vi "Ooi Wei Hong TP065329 Client.vi"() -> ()   [LabVIEW 2023]
uses:
  Control 1.ctl
panel:
  in  "Tab Control":enum32{"Login", "Main"}(tab)
  in  "Request":bool
  out "Password Input":string
  in  "Password":T1
  in  "Reveal":bool
  in  "System Close":bool
  in  "Alarm 1":bool
  in  "Alarm 2":bool
  in  "Alarm 3":bool
  in  "Alarm 4":bool
  in  "Alarm 5":bool
  in  "Alarm 6":bool
  in  "Bypass 1":bool
  in  "Bypass 2":bool
  in  "Bypass 3":bool
  in  "Bypass 4":bool
  in  "Bypass 5":bool
  in  "Bypass 6":bool
  in  "Tamper 1":bool
  in  "Tamper 2":bool
  in  "Tamper 3":bool
  in  "Tamper 4":bool
  in  "Tamper 5":bool
  in  "Tamper 6":bool
  in  "Logout quit":bool
  out "Passcode":string
  # "Vilantguard Technologies Security System"
  # "Alarm Switches"
  # "Bypass Switches"
  # "Tamper Switches"
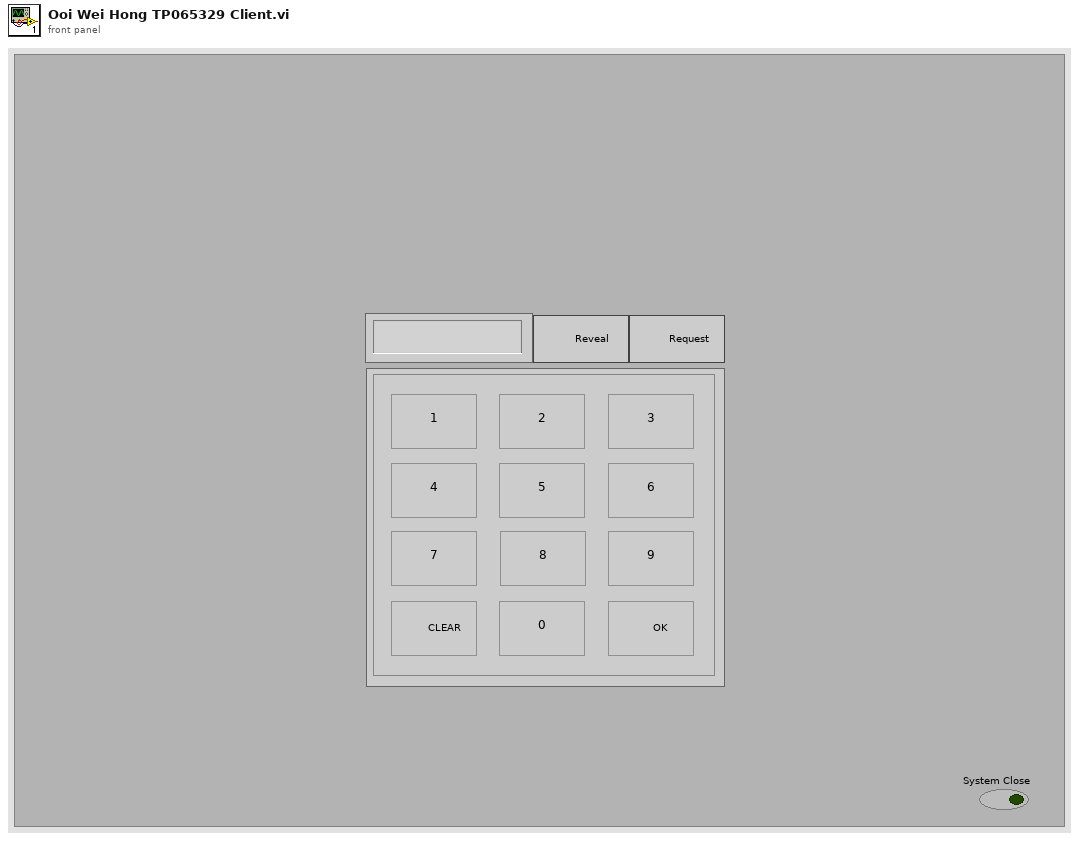
[diagram p1: front panel]
types:
  T1 = cluster{"1":bool, "4":bool, "7":bool, "8":bool, "9":bool, "5":bool, "6":bool, "2":bool, "3":bool, "0":bool, "Previous":bool, "ok":bool}
  T2 = enum8{"Enabled", "Disabled", "Disabled and Grayed Out"}
  T3 = typedef "Control 1.ctl" = enum16{"Init", "Wait", "Zone 1", "Zone 2", "Zone 3", "Zone 4", "Zone 5", "Zone 6"}
  T4 = enum16{"Init", "Wait", "Zone 1", "Zone 2", "Zone 3", "Zone 4", "Zone 5", "Zone 6", "Transmit", "Logging"}
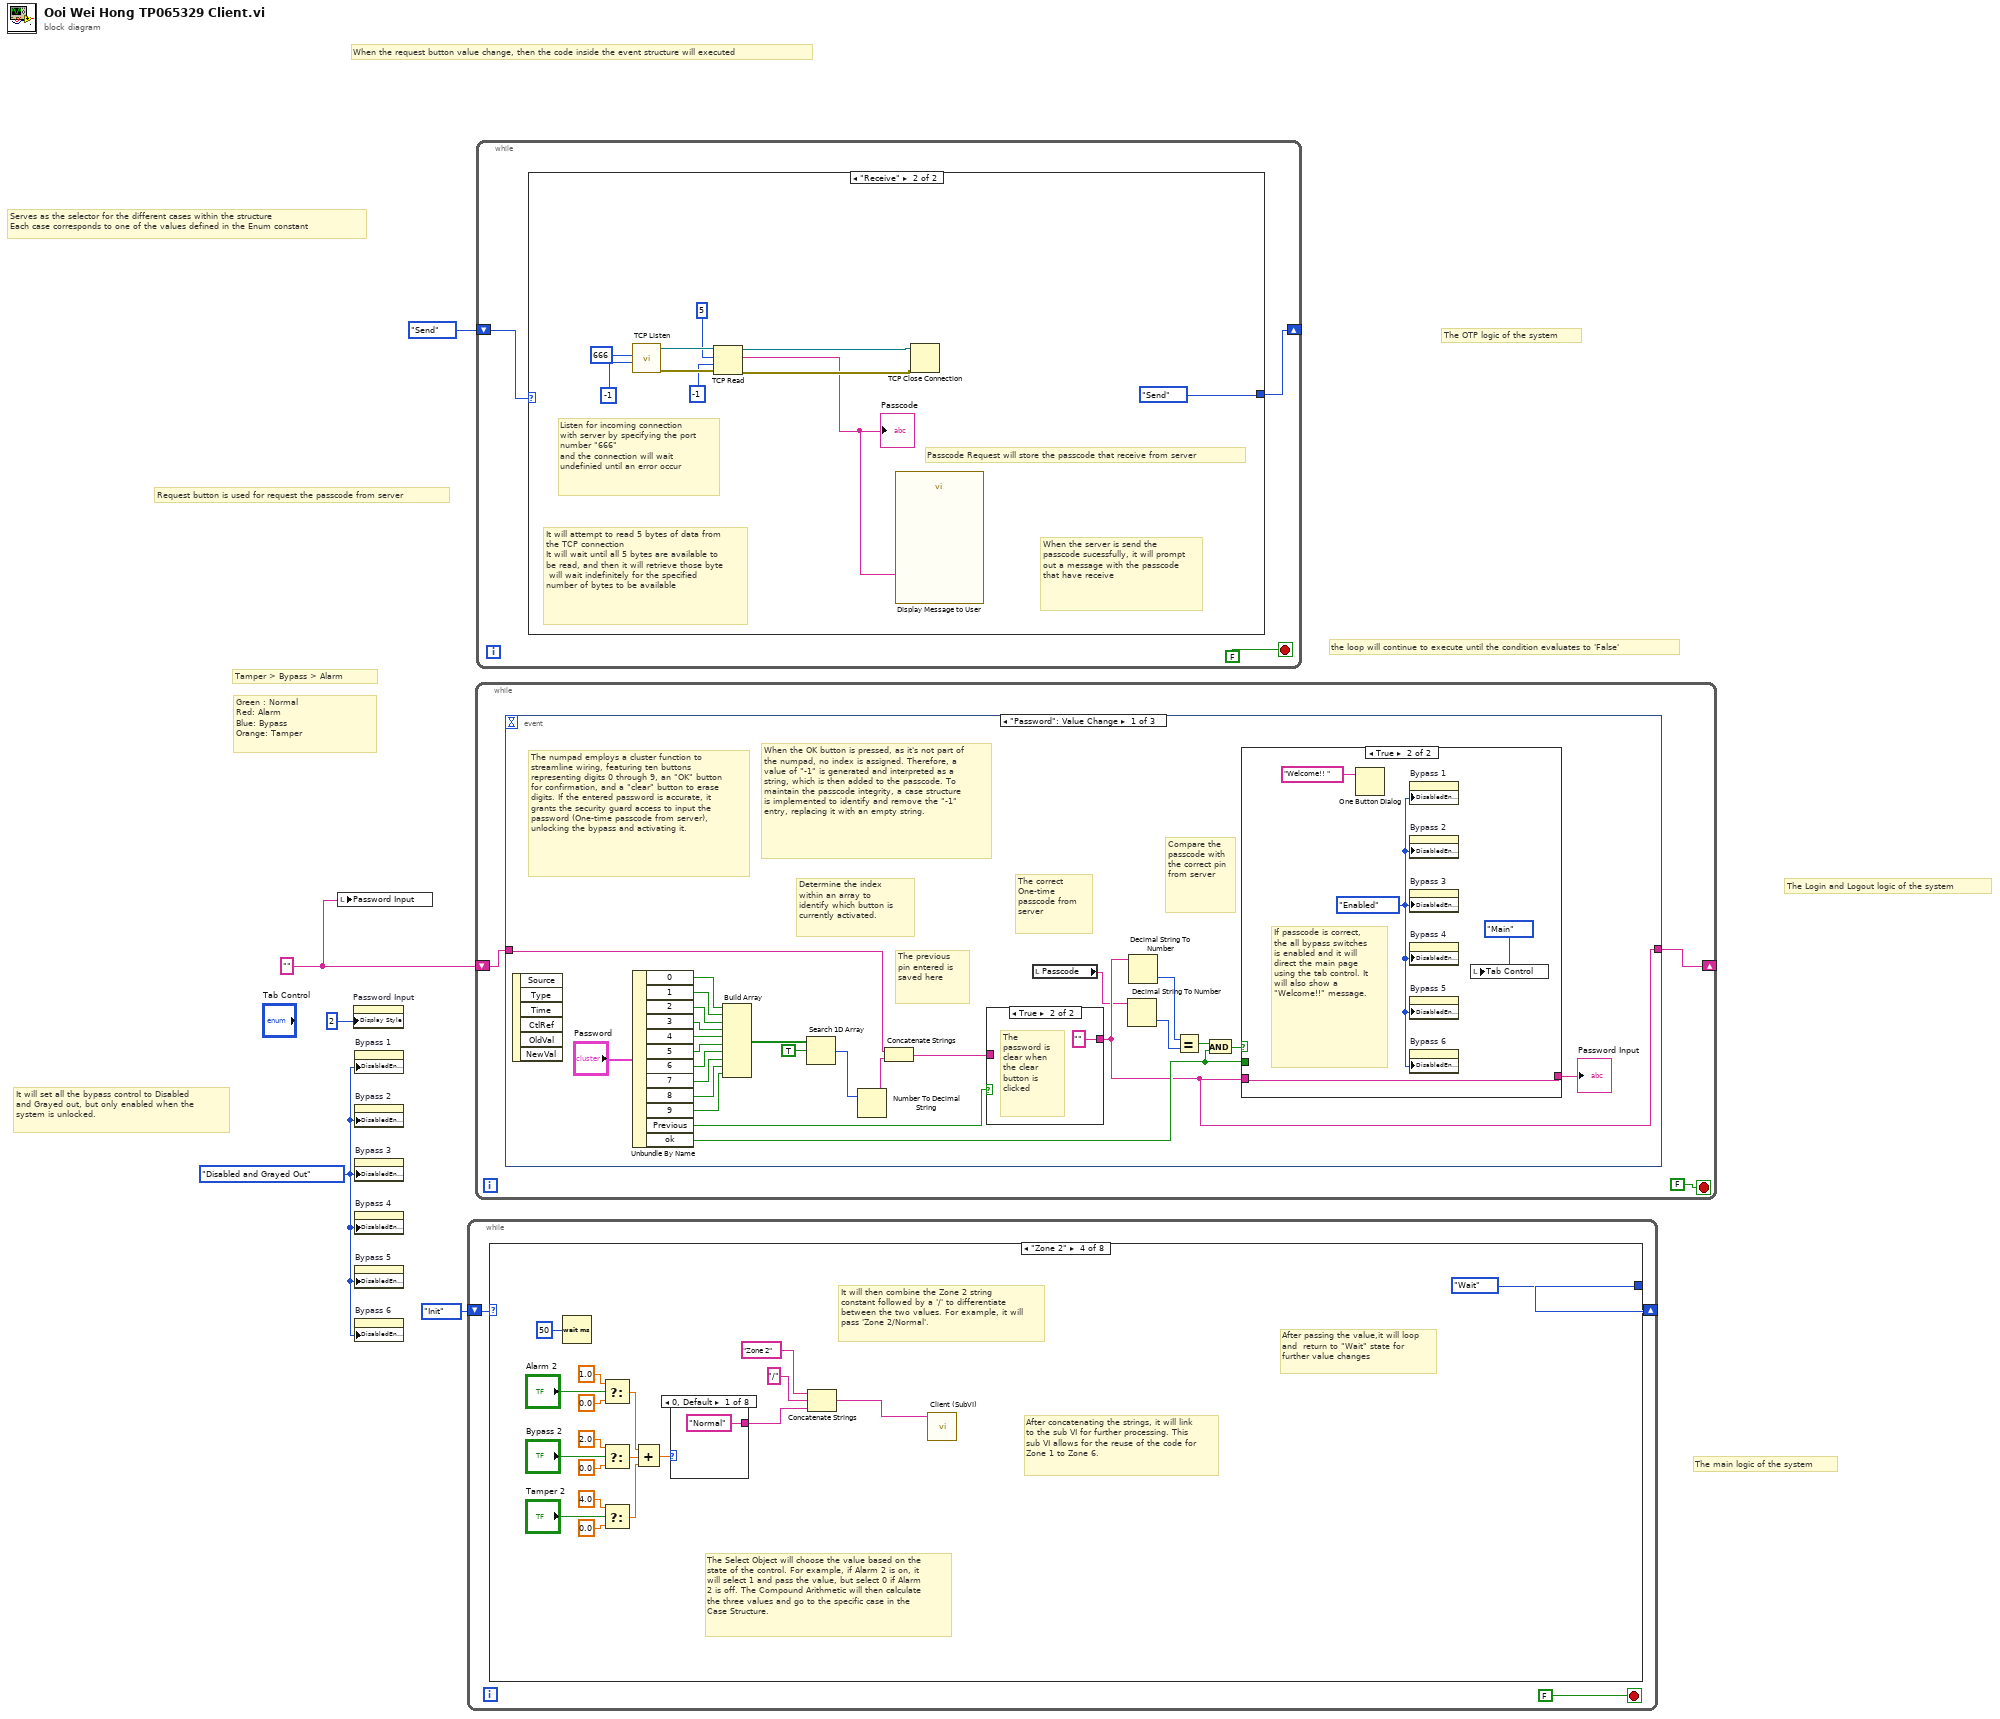
[diagram p0: block diagram]
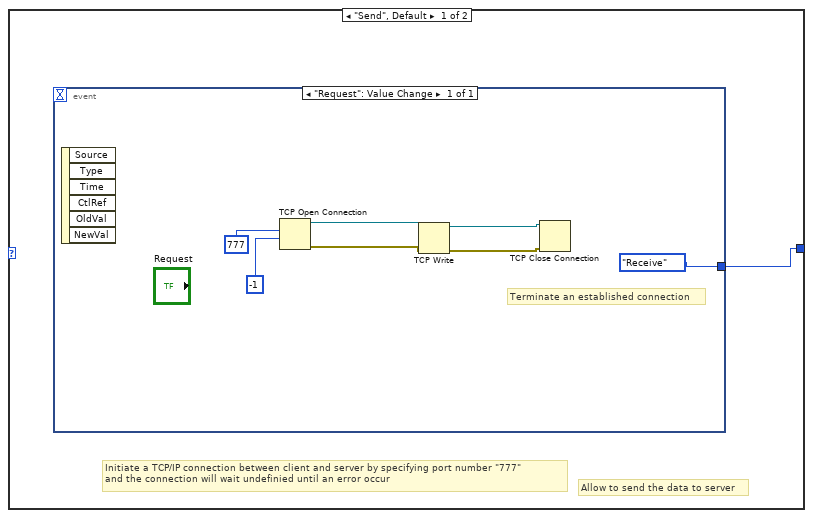
[diagram p2: hidden frame]
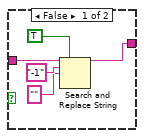
[diagram p3: hidden frame]
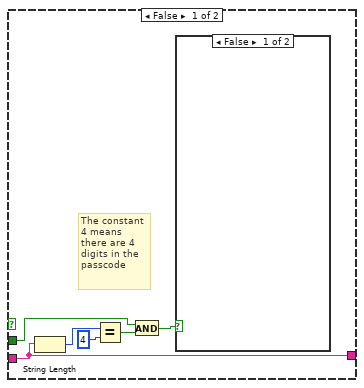
[diagram p4: hidden frame]
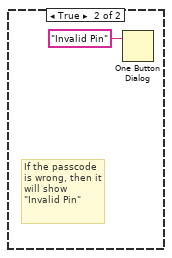
[diagram p5: hidden frame]
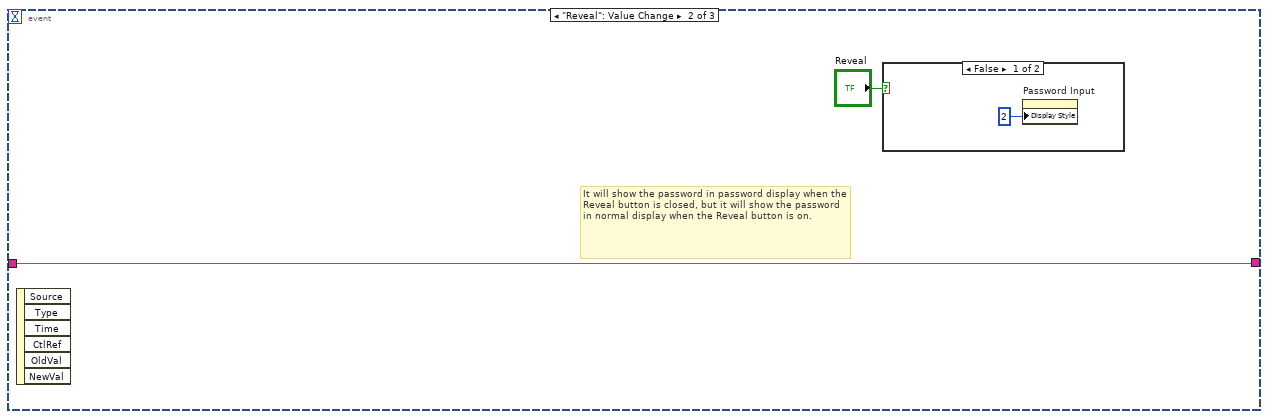
[diagram p6: hidden frame]
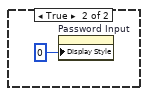
[diagram p7: hidden frame]
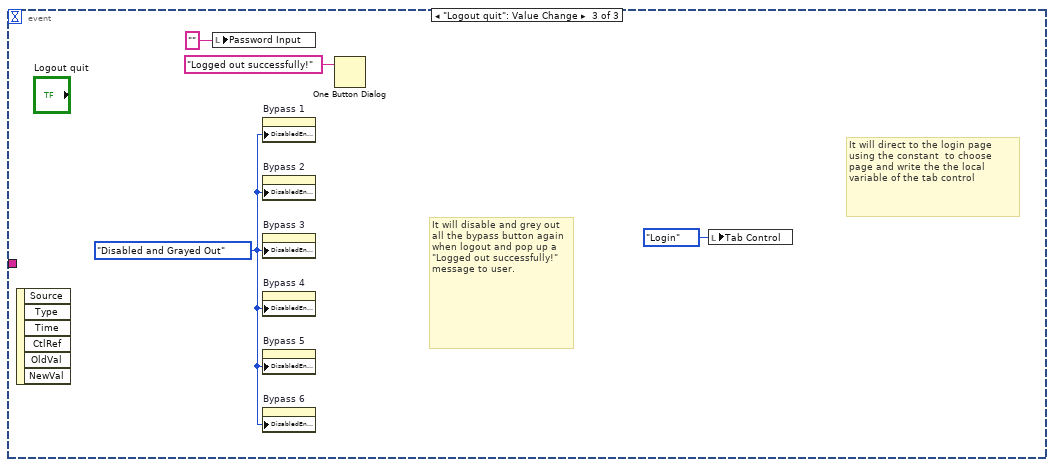
[diagram p8: hidden frame]
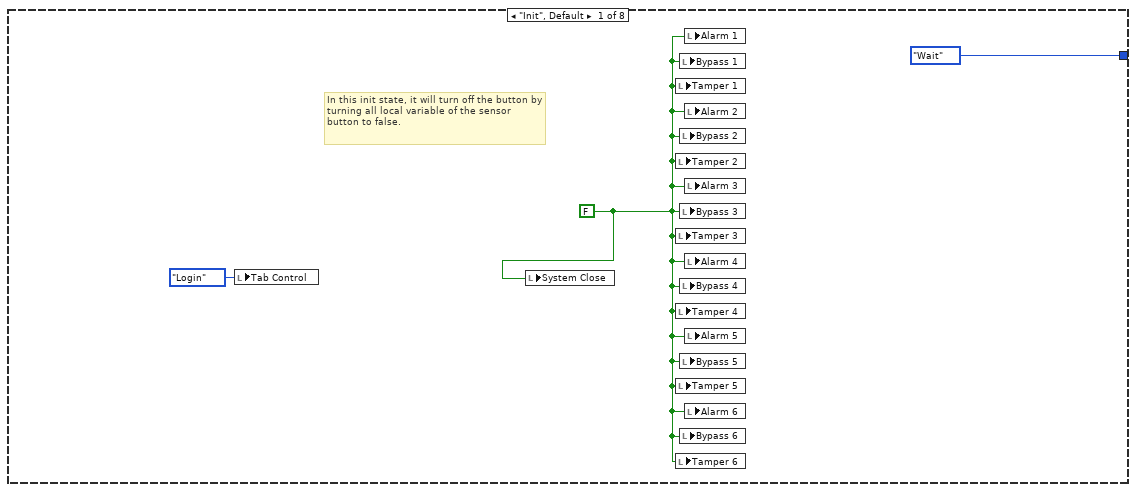
[diagram p9: hidden frame]
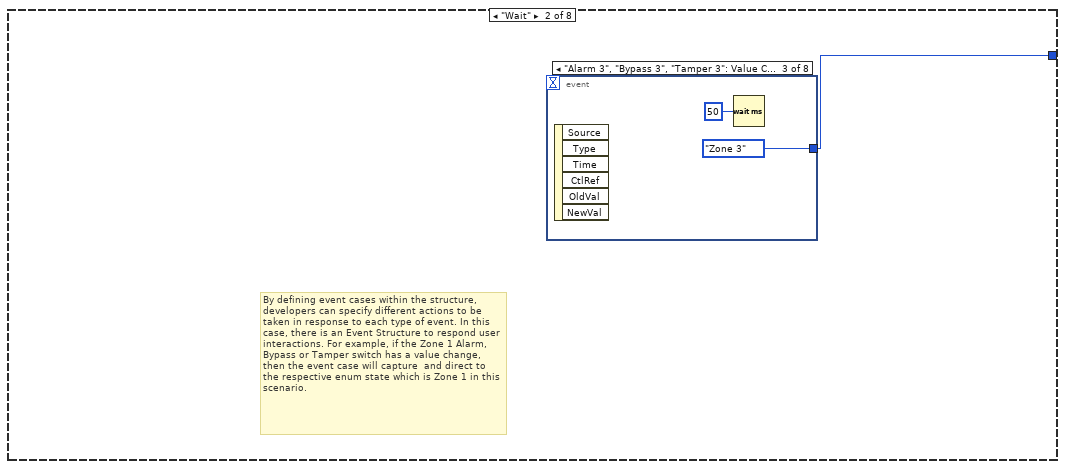
[diagram p10: hidden frame]
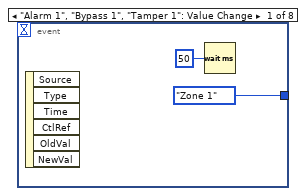
[diagram p11: hidden frame]
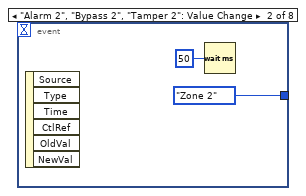
[diagram p12: hidden frame]
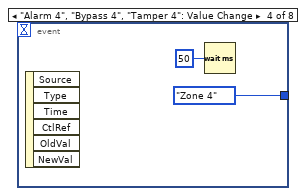
[diagram p13: hidden frame]
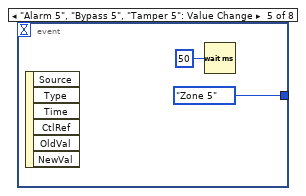
[diagram p14: hidden frame]
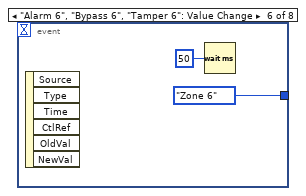
[diagram p15: hidden frame]
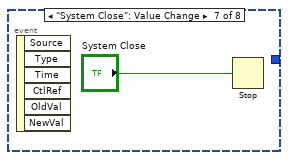
[diagram p16: hidden frame]
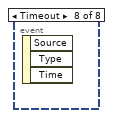
[diagram p17: hidden frame]
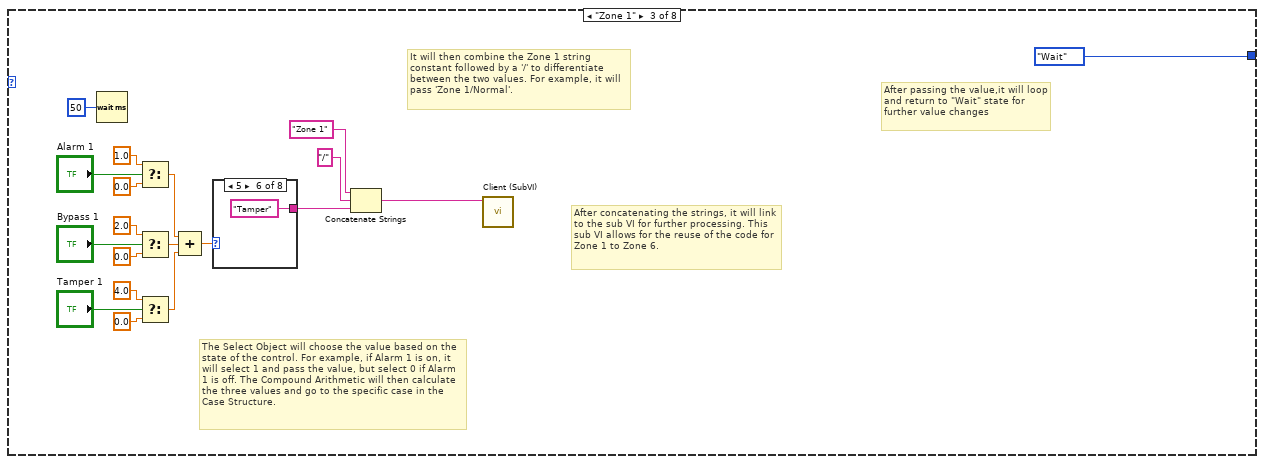
[diagram p18: hidden frame]
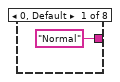
[diagram p19: hidden frame]
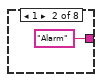
[diagram p20: hidden frame]
diagram:
  w3 = ""
  w4 = T2."Disabled and Grayed Out" ("Disabled")
  # "the loop will continue to execute until the condition evaluates to 'False'"
  # "Request button is used for request the passcode from server"
  # "Serves as the selector for the different cases within the structure\nEach case corresponds to one of the values defined in the Enum constant"
  # "When the request button value change, then the code inside the event structure will executed"
  # "The OTP logic of the system"
  # "The Login and Logout logic of the system"
  # "It will set all the bypass control to Disabled and Grayed out, but only enabled when the system is unlocked."
  # "The main logic of the system"
  # "Green : Normal\nRed: Alarm\nBlue: Bypass\nOrange: Tamper"
  # "Tamper > Bypass > Alarm"
  n1 = local write "Password Input"(w3) -> ()
  n2 = property on="Password Input" class="Str"("Display Style"=u32 2) -> ()  [unwired: 2 in, 2 out]
  n3 = property on="Bypass 1" class="Bool (strict)"("DisabledEnum"=w4) -> ()  [unwired: 2 in, 2 out]
  n4 = property on="Bypass 2" class="Bool (strict)"("DisabledEnum"=w4) -> ()  [unwired: 2 in, 2 out]
  n5 = property on="Bypass 3" class="Bool (strict)"("DisabledEnum"=w4) -> ()  [unwired: 2 in, 2 out]
  n6 = property on="Bypass 4" class="Bool (strict)"("DisabledEnum"=w4) -> ()  [unwired: 2 in, 2 out]
  n7 = property on="Bypass 5" class="Bool (strict)"("DisabledEnum"=w4) -> ()  [unwired: 2 in, 2 out]
  n8 = property on="Bypass 6" class="Bool (strict)"("DisabledEnum"=w4) -> ()  [unwired: 2 in, 2 out]
  n9 = while {
    shift-right: [w8] -> _
    shift-left: Control_1."Init" -> [w7]
    stop <- FALSE stop-if-true
    n10 = case shown="\"Zone 2\"" w7 {
      tunnel: [T4."Wait" w12 Control_1."Wait" Control_1."Wait" Control_1."Wait" Control_1."Wait" Control_1."Wait" Control_1."Wait"] -> w8
      frame "Init", Default {
        w10 = FALSE
        # "In this init state, it will turn off the button by turning all local variable of the sensor button to false."
        n11 = local write "Tab Control"(enum32{"Login", "Main"}."Login" ("Tab Control")) -> ()
        n12 = local write "System Close"(w10) -> ()
        n13 = local write "Tamper 1"(w10) -> ()
        n14 = local write "Tamper 2"(w10) -> ()
        n15 = local write "Tamper 3"(w10) -> ()
        n16 = local write "Tamper 4"(w10) -> ()
        n17 = local write "Tamper 5"(w10) -> ()
        n18 = local write "Tamper 6"(w10) -> ()
        n19 = local write "Bypass 1"(w10) -> ()
        n20 = local write "Bypass 2"(w10) -> ()
        n21 = local write "Bypass 3"(w10) -> ()
        n22 = local write "Bypass 4"(w10) -> ()
        n23 = local write "Bypass 5"(w10) -> ()
        n24 = local write "Bypass 6"(w10) -> ()
        n25 = local write "Alarm 1"(w10) -> ()
        n26 = local write "Alarm 2"(w10) -> ()
        n27 = local write "Alarm 3"(w10) -> ()
        n28 = local write "Alarm 4"(w10) -> ()
        n29 = local write "Alarm 5"(w10) -> ()
        n30 = local write "Alarm 6"(w10) -> ()
      }
      frame "Wait" {
        # "By defining event cases within the structure, developers can specify different actions to be taken in response to each type of event. In this case, there is an Event Structure to respond user interactions. For example, if the Zone 1 Alarm, Bypass or Tamper switch has a value change, then the event case will capture  and direct to the respective enum state which is Zone 1 in this scenario."
        n31 = event shown="[2] \"Alarm 3\", \"Bypass 3\", \"Tamper 3\": Value Change" {
          selector: _ -> [_ _ _ _ _ _ _ _]
          dyn-events: _ -> [_ _ _ _ _ _ _ _]
          timeout: _ -> [_ _ _ _ _ _ _ _]
          tunnel: [Control_1."Zone 1" Control_1."Zone 2" Control_1."Zone 3" Control_1."Zone 4" Control_1."Zone 5" Control_1."Zone 6" _ _] -> w12
          event "Alarm 1", "Bypass 1", "Tamper 1": Value Change {
            n32 = event-data() -> ()  [unwired: 1 in, 6 out]
            n33 = Wait (ms)(milliseconds to wait=u32 50) -> ()  [unwired: 1 out]
          }
          event "Alarm 2", "Bypass 2", "Tamper 2": Value Change {
            n34 = event-data() -> ()  [unwired: 1 in, 6 out]
            n35 = Wait (ms)(milliseconds to wait=u32 50) -> ()  [unwired: 1 out]
          }
          event "Alarm 3", "Bypass 3", "Tamper 3": Value Change {
            n36 = event-data() -> ()  [unwired: 1 in, 6 out]
            n37 = Wait (ms)(milliseconds to wait=u32 50) -> ()  [unwired: 1 out]
          }
          event "Alarm 4", "Bypass 4", "Tamper 4": Value Change {
            n38 = event-data() -> ()  [unwired: 1 in, 6 out]
            n39 = Wait (ms)(milliseconds to wait=u32 50) -> ()  [unwired: 1 out]
          }
          event "Alarm 5", "Bypass 5", "Tamper 5": Value Change {
            n40 = event-data() -> ()  [unwired: 1 in, 6 out]
            n41 = Wait (ms)(milliseconds to wait=u32 50) -> ()  [unwired: 1 out]
          }
          event "Alarm 6", "Bypass 6", "Tamper 6": Value Change {
            n42 = event-data() -> ()  [unwired: 1 in, 6 out]
            n43 = Wait (ms)(milliseconds to wait=u32 50) -> ()  [unwired: 1 out]
          }
          event "System Close": Value Change {
            n44 = event-data() -> ()  [unwired: 1 in, 6 out]
            n45 = Stop(stop? (T)="System Close") -> ()
          }
          event Timeout {
            n46 = event-data() -> ()  [unwired: 1 in, 3 out]
          }
        }
      }
      frame "Zone 1" {
        # "After concatenating the strings, it will link to the sub VI for further processing. This sub VI allows for the reuse of the code for Zone 1 to Zone 6."
        # "After passing the value,it will loop and return to \"Wait\" state for further value changes"
        # "It will then combine the Zone 1 string constant followed by a '/' to differentiate between the two values. For example, it will pass 'Zone 1/Normal'."
        # "The Select Object will choose the value based on the state of the control. For example, if Alarm 1 is on, it will select 1 and pass the value, but select 0 if Alarm 1 is off. The Compound Arithmetic will then calculate the three values and go to the specific case in the Case Structure."
        n47 = Wait (ms)(milliseconds to wait=u32 50) -> ()  [unwired: 1 out]
        n48 = Select(t=1.0, s="Alarm 1", f=0.0) -> (s? t:f=w41:dbl)
        n49 = Select(t=2.0, s="Bypass 1", f=0.0) -> (s? t:f=w42:dbl)
        n50 = Select(t=4.0, s="Tamper 1", f=0.0) -> (s? t:f=w43:dbl)
        n51 = Compound Arithmetic op=ADD(w41, w42, w43) -> (w44:dbl)
        n52 = case shown="5" w44 {
          tunnel: ["Normal" "Alarm" "Bypass" "Bypass" "Tamper" "Tamper" "Tamper" "Tamper"] -> w28
          frame 0, Default {
          }
          frame 1 {
          }
          frame 2 {
          }
          frame 3 {
          }
          frame 4 {
          }
          frame 5 {
          }
          frame 6 {
          }
          frame 7 {
          }
        }
        n53 = Concatenate Strings "Concatenate Strings"("Zone 1", "/", w28) -> (w27:string)
        n54 = call "Client (SubVI).vi"("String"=w27) -> ()  [unwired: 11 in]
      }
      frame "Zone 2" {
        # "After concatenating the strings, it will link to the sub VI for further processing. This sub VI allows for the reuse of the code for Zone 1 to Zone 6."
        # "After passing the value,it will loop and  return to \"Wait\" state for further value changes"
        # "The Select Object will choose the value based on the state of the control. For example, if Alarm 2 is on, it will select 1 and pass the value, but select 0 if Alarm 2 is off. The Compound Arithmetic will then calculate the three values and go to the specific case in the Case Structure."
        # "It will then combine the Zone 2 string constant followed by a '/' to differentiate between the two values. For example, it will pass 'Zone 2/Normal'."
        n55 = Wait (ms)(milliseconds to wait=u32 50) -> ()  [unwired: 1 out]
        n56 = Select(t=1.0, s="Alarm 2", f=0.0) -> (s? t:f=w68:dbl)
        n57 = Select(t=2.0, s="Bypass 2", f=0.0) -> (s? t:f=w69:dbl)
        n58 = Select(t=4.0, s="Tamper 2", f=0.0) -> (s? t:f=w70:dbl)
        n59 = Compound Arithmetic op=ADD(w68, w69, w70) -> (w71:dbl)
        n60 = case shown="0, Default" w71 {
          tunnel: ["Normal" "Alarm" "Bypass" "Bypass" "Tamper" "Tamper" "Tamper" "Tamper"] -> w58
          frame 0, Default {
          }
          frame 1 {
          }
          frame 2 {
          }
          frame 3 {
          }
          frame 4 {
          }
          frame 5 {
          }
          frame 6 {
          }
          frame 7 {
          }
        }
        n61 = Concatenate Strings "Concatenate Strings"("Zone 2", "/", w58) -> (w53:string)
        n62 = call "Client (SubVI).vi"("String"=w53) -> ()  [unwired: 11 in]
      }
      frame "Zone 3" {
        # "After concatenating the strings, it will link to the sub VI for further processing. This sub VI allows for the reuse of the code for Zone 1 to Zone 6."
        # "It will then combine the Zone 3 string constant followed by a '/' to differentiate between the two values. For example, it will pass 'Zone 3/Normal'."
        # "The Select Object will choose the value based on the state of the control. For example, if Alarm 3 is on, it will select 1 and pass the value, but select 0 if Alarm 3 is off. The Compound Arithmetic will then calculate the three values and go to the specific case in the Case Structure."
        # "After passing the value,it will loop and  return to \"Wait\" state for further value changes"
        n63 = Wait (ms)(milliseconds to wait=u32 50) -> ()  [unwired: 1 out]
        n64 = Select(t=1.0, s="Alarm 3", f=0.0) -> (s? t:f=w93:dbl)
        n65 = Select(t=2.0, s="Bypass 3", f=0.0) -> (s? t:f=w94:dbl)
        n66 = Select(t=4.0, s="Tamper 3", f=0.0) -> (s? t:f=w95:dbl)
        n67 = Compound Arithmetic op=ADD(w93, w94, w95) -> (w96:dbl)
        n68 = case shown="0, Default" w96 {
          tunnel: ["Normal" "Alarm" "Bypass" "Bypass" "Tamper" "Tamper" "Tamper" "Tamper"] -> w84
          frame 0, Default {
          }
          frame 1 {
          }
          frame 2 {
          }
          frame 3 {
          }
          frame 4 {
          }
          frame 5 {
          }
          frame 6 {
          }
          frame 7 {
          }
        }
        n69 = Concatenate Strings "Concatenate Strings"("Zone 3", "/", w84) -> (w80:string)
        n70 = call "Client (SubVI).vi"("String"=w80) -> ()  [unwired: 11 in]
      }
      frame "Zone 4" {
        # "After concatenating the strings, it will link to the sub VI for further processing. This sub VI allows for the reuse of the code for Zone 1 to Zone 6."
        # "After passing the value,it will loop and  return to \"Wait\" state for further value changes"
        # "The Select Object will choose the value based on the state of the control. For example, if Alarm 4 is on, it will select 1 and pass the value, but select 0 if Alarm 4 is off. The Compound Arithmetic will then calculate the three values and go to the specific case in the Case Structure."
        # "It will then combine the Zone 4 string constant followed by a '/' to differentiate between the two values. For example, it will pass 'Zone 4/Normal'."
        n71 = Wait (ms)(milliseconds to wait=u32 50) -> ()  [unwired: 1 out]
        n72 = Select(t=1.0, s="Alarm 4", f=0.0) -> (s? t:f=w120:dbl)
        n73 = Select(t=2.0, s="Bypass 4", f=0.0) -> (s? t:f=w121:dbl)
        n74 = Select(t=4.0, s="Tamper 4", f=0.0) -> (s? t:f=w122:dbl)
        n75 = Compound Arithmetic op=ADD(w120, w121, w122) -> (w123:dbl)
        n76 = case shown="0, Default" w123 {
          tunnel: ["Normal" "Alarm" "Bypass" "Bypass" "Tamper" "Tamper" "Tamper" "Tamper"] -> w111
          frame 0, Default {
          }
          frame 1 {
          }
          frame 2 {
          }
          frame 3 {
          }
          frame 4 {
          }
          frame 5 {
          }
          frame 6 {
          }
          frame 7 {
          }
        }
        n77 = Concatenate Strings "Concatenate Strings"("Zone 4", "/", w111) -> (w107:string)
        n78 = call "Client (SubVI).vi"("String"=w107) -> ()  [unwired: 11 in]
      }
      frame "Zone 5" {
        # "After concatenating the strings, it will link to the sub VI for further processing. This sub VI allows for the reuse of the code for Zone 1 to Zone 6."
        # "It will then combine the Zone 5 string constant followed by a '/' to differentiate between the two values. For example, it will pass 'Zone 5/Normal'."
        # "The Select Object will choose the value based on the state of the control. For example, if Alarm 5 is on, it will select 1 and pass the value, but select 0 if Alarm 5 is off. The Compound Arithmetic will then calculate the three values and go to the specific case in the Case Structure."
        # "After passing the value,it will loop and  return to \"Wait\" state for further value changes"
        n79 = Wait (ms)(milliseconds to wait=u32 50) -> ()  [unwired: 1 out]
        n80 = Select(t=1.0, s="Alarm 5", f=0.0) -> (s? t:f=w147:dbl)
        n81 = Select(t=2.0, s="Bypass 5", f=0.0) -> (s? t:f=w148:dbl)
        n82 = Select(t=4.0, s="Tamper 5", f=0.0) -> (s? t:f=w149:dbl)
        n83 = Compound Arithmetic op=ADD(w147, w148, w149) -> (w150:dbl)
        n84 = case shown="0, Default" w150 {
          tunnel: ["Normal" "Alarm" "Bypass" "Bypass" "Tamper" "Tamper" "Tamper" "Tamper"] -> w138
          frame 0, Default {
          }
          frame 1 {
          }
          frame 2 {
          }
          frame 3 {
          }
          frame 4 {
          }
          frame 5 {
          }
          frame 6 {
          }
          frame 7 {
          }
        }
        n85 = Concatenate Strings "Concatenate Strings"("Zone 5", "/", w138) -> (w134:string)
        n86 = call "Client (SubVI).vi"("String"=w134) -> ()  [unwired: 11 in]
      }
      frame "Zone 6" {
        # "After concatenating the strings, it will link to the sub VI for further processing. This sub VI allows for the reuse of the code for Zone 1 to Zone 6."
        # "After passing the value,it will loop and  return to \"Wait\" state for further value changes"
        # "The Select Object will choose the value based on the state of the control. For example, if Alarm 6 is on, it will select 1 and pass the value, but select 0 if Alarm 6 is off. The Compound Arithmetic will then calculate the three values and go to the specific case in the Case Structure."
        # "It will then combine the Zone 6 string constant followed by a '/' to differentiate between the two values. For example, it will pass 'Zone 6/Normal'."
        n87 = Select(t=1.0, s="Alarm 6", f=0.0) -> (s? t:f=w174:dbl)
        n88 = Select(t=2.0, s="Bypass 6", f=0.0) -> (s? t:f=w175:dbl)
        n89 = Select(t=4.0, s="Tamper 6", f=0.0) -> (s? t:f=w176:dbl)
        n90 = Wait (ms)(milliseconds to wait=u32 50) -> ()  [unwired: 1 out]
        n91 = Compound Arithmetic op=ADD(w174, w175, w176) -> (w177:dbl)
        n92 = case shown="0, Default" w177 {
          tunnel: ["Normal" "Alarm" "Bypass" "Bypass" "Tamper" "Tamper" "Tamper" "Tamper"] -> w165
          frame 0, Default {
          }
          frame 1 {
          }
          frame 2 {
          }
          frame 3 {
          }
          frame 4 {
          }
          frame 5 {
          }
          frame 6 {
          }
          frame 7 {
          }
        }
        n93 = Concatenate Strings "Concatenate Strings"("Zone 6", "/", w165) -> (w161:string)
        n94 = call "Client (SubVI).vi"("String"=w161) -> ()  [unwired: 11 in]
      }
    }
  }
  n95 = while {
    shift-right: [w188] -> _
    shift-left: w3 -> [w190]
    stop <- FALSE stop-if-true
    n96 = event shown="[0] \"Password\": Value Change" {
      selector: _ -> [_ _ _]
      dyn-events: _ -> [_ _ _]
      timeout: _ -> [_ _ _]
      tunnel: w190 -> [w201 w234 _]
      tunnel: [w194 w234 _] -> w188
      event "Password": Value Change {
        # "When the OK button is pressed, as it's not part of the numpad, no index is assigned. Therefore, a value of \"-1\" is generated and interpreted as a string, which is then added to the passcode. To maintain the passcode integrity, a case structure is implemented to identify and remove the \"-1\" entry, replacing it with an empty string."
        # "The previous pin entered is saved here"
        # "The correct One-time passcode from server"
        # "Compare the passcode with the correct pin from server"
        # "Determine the index within an array to identify which button is currently activated."
        # "The numpad employs a cluster function to streamline wiring, featuring ten buttons representing digits 0 through 9, an \"OK\" button for confirmation, and a \"clear\" button to erase digits. If the entered password is accurate, it grants the security guard access to input the password (One-time passcode from server), unlocking the bypass and activating it."
        n97 = event-data() -> ()  [unwired: 1 in, 6 out]
        n98 = Unbundle By Name "Unbundle By Name"("Password") -> ("0"=w215:bool, "1"=w214:bool, "2"=w213:bool, "3"=w212:bool, "4"=w211:bool, "5"=w210:bool, "6"=w209:bool, "7"=w208:bool, "8"=w207:bool, "9"=w206:bool, "Previous"=w198:bool, "ok"=w195:bool)
        n99 = Build Array(w215, w214, w213, w212, w211, w210, w209, w208, w207, w206) -> (w205:bool[])
        n100 = Search 1D Array(1D array=w205, element=TRUE) -> (index of element=w204:i32)  [unwired: 1 in]
        n101 = Number To Decimal String(number=w204) -> (decimal integer string=w202:string)  [unwired: 1 in]
        n102 = Concatenate Strings "Concatenate Strings"(w201, w202) -> (w199:string)
        n103 = case shown="True" w198 {
          tunnel: w199 -> [w221 _]
          tunnel: [w218 ""] -> w194
          frame False {
            n104 = Search and Replace String(replace all?=TRUE, input string=w221, search string="-1", replace string="" ("replace string (\"\")")) -> (result string=w218:string)  [unwired: 4 in, 3 out]
          }
          frame True {
            # "The password is clear when the clear button is clicked"
          }
        }
        n105 = local read "Passcode"() -> (w192:string)
        n106 = Decimal String To Number(string=w192) -> (number=w191:i32)  [unwired: 2 in, 1 out]
        n107 = Decimal String To Number(string=w194) -> (number=w193:i32)  [unwired: 2 in, 1 out]
        n108 = Equal?(x=w193, y=w191) -> (x = y?=w196:bool)
        n109 = And(x=w196, y=w195) -> (x .and. y?=w200:bool)
        n110 = case shown="True" w200 {
          tunnel: w194 -> [w226 w232]
          tunnel: [w226 w232] -> w197
          tunnel: w195 -> [w228 _]
          frame False {
            # "The constant 4 means there are 4 digits in the passcode"
            n111 = String Length(string=w226) -> (length=w225:i32)
            n112 = Equal?(x=w225, y=4) -> (x = y?=w223:bool)
            n113 = And(x=w228, y=w223) -> (x .and. y?=w227:bool)
            n114 = case shown="False" w227 {
              frame False {
              }
              frame True {
                # "If the passcode is wrong, then it will show \"Invalid Pin\""
                n115 = One Button Dialog(message="Invalid Pin") -> ()  [unwired: 1 in, 1 out]
              }
            }
          }
          frame True {
            w230 = T2."Enabled" ("Disabled")
            # "If passcode is correct, the all bypass switches is enabled and it will direct the main page using the tab control. It will also show a \"Welcome!!\" message."
            n116 = One Button Dialog(message="Welcome!! ") -> ()  [unwired: 1 in, 1 out]
            n117 = property on="Bypass 1" class="Bool (strict)"("DisabledEnum"=w230) -> ()  [unwired: 2 in, 2 out]
            n118 = property on="Bypass 2" class="Bool (strict)"("DisabledEnum"=w230) -> ()  [unwired: 2 in, 2 out]
            n119 = property on="Bypass 3" class="Bool (strict)"("DisabledEnum"=w230) -> ()  [unwired: 2 in, 2 out]
            n120 = property on="Bypass 4" class="Bool (strict)"("DisabledEnum"=w230) -> ()  [unwired: 2 in, 2 out]
            n121 = property on="Bypass 5" class="Bool (strict)"("DisabledEnum"=w230) -> ()  [unwired: 2 in, 2 out]
            n122 = property on="Bypass 6" class="Bool (strict)"("DisabledEnum"=w230) -> ()  [unwired: 2 in, 2 out]
            n123 = local write "Tab Control"(enum32{"Login", "Main"}."Main" ("Tab Control")) -> ()
          }
        }
        "Password Input" <- w197
      }
      event "Reveal": Value Change {
        # "It will show the password in password display when the Reveal button is closed, but it will show the password in normal display when the Reveal button is on."
        n124 = event-data() -> ()  [unwired: 1 in, 6 out]
        n125 = case shown="False" "Reveal" {
          frame False {
            n126 = property on="Password Input" class="Str"("Display Style"=u32 2) -> ()  [unwired: 2 in, 2 out]
          }
          frame True {
            n127 = property on="Password Input" class="Str"("Display Style"=u32 0) -> ()  [unwired: 2 in, 2 out]
          }
        }
      }
      event "Logout quit": Value Change {
        w238 = T2."Disabled and Grayed Out" ("Disabled")
        # "It will direct to the login page using the constant  to choose page and write the the local variable of the tab control"
        # "It will disable and grey out all the bypass button again when logout and pop up a \"Logged out successfully!\" message to user."
        n128 = event-data() -> ()  [unwired: 1 in, 6 out]
        n129 = local write "Password Input"("") -> ()
        n130 = property on="Bypass 1" class="Bool (strict)"("DisabledEnum"=w238) -> ()  [unwired: 2 in, 2 out]
        n131 = property on="Bypass 2" class="Bool (strict)"("DisabledEnum"=w238) -> ()  [unwired: 2 in, 2 out]
        n132 = property on="Bypass 3" class="Bool (strict)"("DisabledEnum"=w238) -> ()  [unwired: 2 in, 2 out]
        n133 = property on="Bypass 4" class="Bool (strict)"("DisabledEnum"=w238) -> ()  [unwired: 2 in, 2 out]
        n134 = property on="Bypass 5" class="Bool (strict)"("DisabledEnum"=w238) -> ()  [unwired: 2 in, 2 out]
        n135 = property on="Bypass 6" class="Bool (strict)"("DisabledEnum"=w238) -> ()  [unwired: 2 in, 2 out]
        n136 = One Button Dialog(message="Logged out successfully!") -> ()  [unwired: 1 in, 1 out]
        n137 = local write "Tab Control"(enum32{"Login", "Main"}."Login" ("Tab Control")) -> ()
      }
    }
  }
  n138 = while {
    shift-right: [w243] -> _
    shift-left: enum16{"Send", "Receive"}."Send" -> [w242]
    stop <- FALSE stop-if-true
    n139 = case shown="\"Receive\"" w242 {
      tunnel: [w245 enum16{"Send", "Receive"}."Send"] -> w243
      frame "Send", Default {
        # "Allow to send the data to server"
        # "Initiate a TCP/IP connection between client and server by specifying port number \"777\" \nand the connection will wait undefinied until an error occur"
        n140 = event shown="[0] \"Request\": Value Change" {
          selector: _ -> [_]
          dyn-events: _ -> [_]
          timeout: _ -> [_]
          tunnel: [enum16{"Send", "Receive"}."Receive"] -> w245
          event "Request": Value Change {
            # "Terminate an established connection"
            n141 = event-data() -> ()  [unwired: 1 in, 6 out]
            n142 = TCP Open Connection(remote port or service name=u16 777, timeout ms (60000)=-1) -> (connection ID=w249:refnum<k5>, error out=w252:errorcluster)  [unwired: 3 in]
            n143 = TCP Write(connection ID=w249, error in (no error)=w252) -> (connection ID out=w250:refnum<k5>, error out=w251:errorcluster)  [unwired: 2 in, 1 out]
            n144 = TCP Close Connection(connection ID=w250, error in (no error)=w251) -> ()  [unwired: 1 in, 2 out]
          }
        }
      }
      frame "Receive" {
        # "It will attempt to read 5 bytes of data from the TCP connection\nIt will wait until all 5 bytes are available to be read, and then it will retrieve those byte\n will wait indefinitely for the specified number of bytes to be available"
        # "Listen for incoming connection with server by specifying the port number \"666\" \nand the connection will wait undefinied until an error occur"
        # "When the server is send the passcode sucessfully, it will prompt out a message with the passcode that have receive"
        # "Passcode Request will store the passcode that receive from server"
        n145 = call <vilib>:"TCP Listen.vi"("timeout ms (wait forever: -1)"=-1, "port"=u16 666) -> ("error out"=w261:errorcluster, "connection ID"=w262:refnum<k5>)  [unwired: 5 in, 3 out]
        n146 = TCP Read(connection ID=w262, bytes to read=5, error in (no error)=w261, 9:-1 ("timeout ms (25000)")) -> (connection ID out=w258:refnum<k5>, data out=w253:string, error out=w257:errorcluster)  [unwired: 1 in]
        "Passcode" <- w253
        n147 = call "Display Message to User"("Message"=w253) -> ()  [unwired: 9 in, 2 out]
        n148 = TCP Close Connection(connection ID=w258, error in (no error)=w257) -> ()  [unwired: 1 in, 2 out]
      }
    }
  }
